vi "GETPINSTATUS.vi"(8 "error in (no error)":errorcluster, 9 "pin":dbl, 10 "Port":dbl, 11 "Arduino in":refnum<class "Arduino.lvclass">) -> (0 "error out":errorcluster, 3 "Arduino out":refnum<class "Arduino.lvclass">)   [LabVIEW 2019, in "Arduino.lvclass"]
uses:
  Arduino.lvclass
  Arduino.lvclass/Arduino.ctl
  9b87b02a-03e6-410b-895e-ea7083fa135d.vi
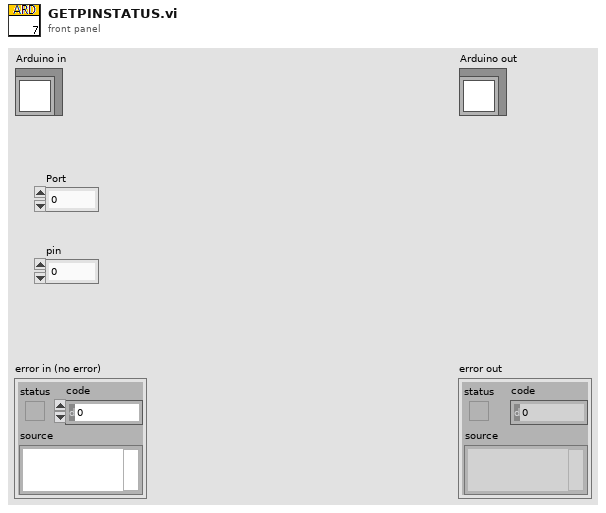
[diagram p1: front panel]
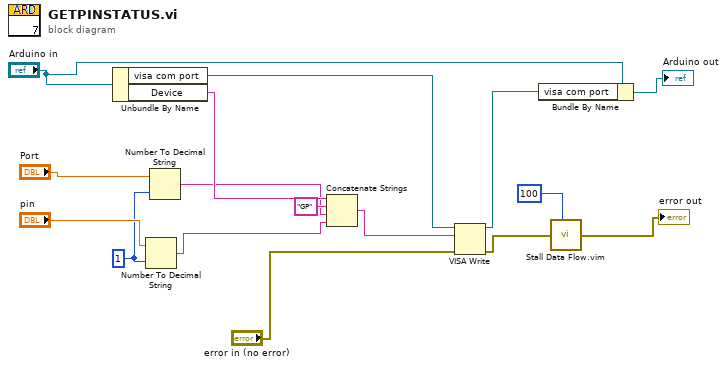
[diagram p0: block diagram]
diagram:
  w14 = i16 1 ("width (-)")
  n1 = Unbundle By Name("Arduino in") -> ("visa com port"=w2:refnum<visa-resource-name>, "Device"=w13:string)
  n2 = Number To Decimal String(number="pin", width (-)=w14) -> (decimal integer string=w3:string)
  n3 = Number To Decimal String(number="Port", width (-)=w14) -> (decimal integer string=w11:string)
  n4 = Concatenate Strings(w13, "GP" ("string"), w11, w3) -> (w10:string)
  n5 = VISA Write(VISA resource name=w2, write buffer=w10, error in (no error)="error in (no error)") -> (VISA resource name out=w4:refnum<visa-resource-name>, error out=w9:errorcluster)  [unwired: 1 out]
  n6 = Bundle By Name(cluster="Arduino in", "visa com port"=w4) -> (→"Arduino out":refnum<class "Arduino.lvclass">)
  n7 = call "Stall Data Flow.vim"("value in"=w9, "milliseconds to wait"=u32 100) -> ("value out"=→"error out":errorcluster)  [unwired: 1 out]
